vi "fgv_gps_config.vi"(7 "cmd":enum16{"read", "write"}(ring), 8 "error in":errorcluster, 11 "cfg":T1={"Port"="COM5", "heading select"="NARROW_INT", "mode select"=["INS_RTKFIXED", "INS_RTKFLOAT"]}) -> (0 "error out":errorcluster, 3 "cfg out":T1={"Port"="COM5", "heading select"="NARROW_INT", "mode select"=["INS_RTKFIXED", "INS_RTKFLOAT"]})   [LabVIEW 2019]
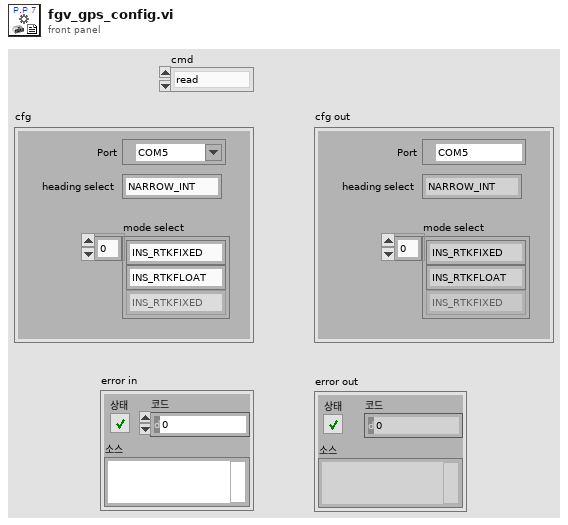
[diagram p1: front panel]
types:
  T1 = cluster{"Port":refnum<visa-resource-name>, "heading select":string, "mode select":string[]}
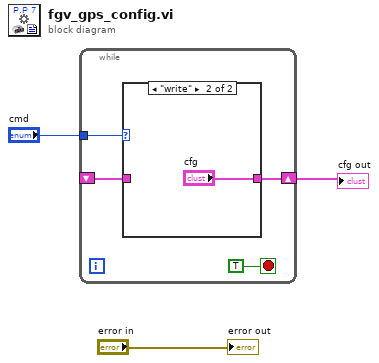
[diagram p0: block diagram]
diagram:
  n1 = while {
    tunnel: "cmd" -> [w6]
    shift-right: [w5] -> w1
    shift-left: _ -> [w4]
    stop <- TRUE stop-if-true
    n2 = case shown="\"write\"" w6 {
      tunnel: [w8 "cfg"] -> w5
      tunnel: w4 -> [w8 _]
      frame "read", Default {
      }
      frame "write" {
      }
    }
  }
  "cfg out" <- w1
  "error out" <- "error in"
